vi "KE622x -- 2182 -A Set Digital Filter Type.vi"(0 "622x Resource In":refnum<visa-resource-name>, 1 "Check For SCPI Errors? (T)":bool=TRUE, 7 "Filter Type":T1=enum."Repeat", 11 "error in (no error)":errorcluster) -> (4 "622x Resource Out (dupl)":refnum<visa-resource-name>, 15 "error out":errorcluster)   [LabVIEW 2019, in "Keithley 622x.lvlib"]
uses:
  Keithley 622x.lvlib
  Typedefs/KE2182 -- Filter Type.ctl
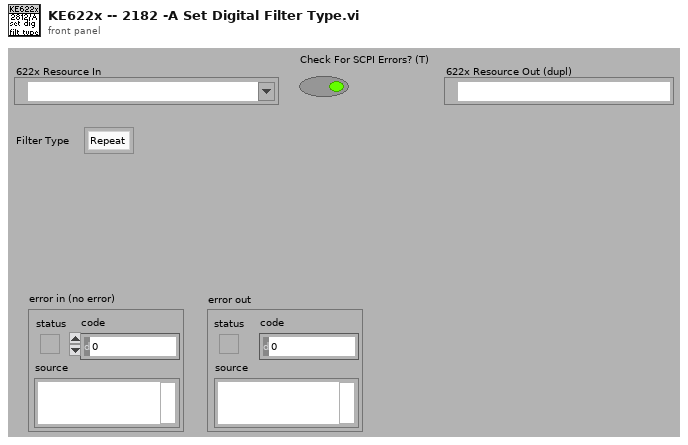
[diagram p1: front panel]
types:
  T1 = typedef "Keithley 622x.lvlib/KE2182 -- Filter Type.ctl" = enum16{"Moving", "Repeat"}
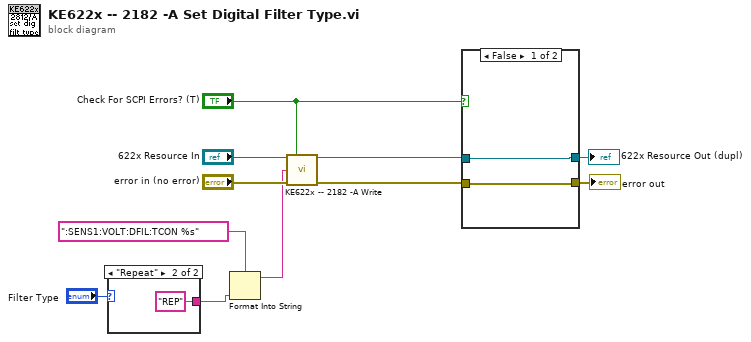
[diagram p0: block diagram]
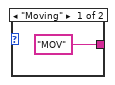
[diagram p2: hidden frame]
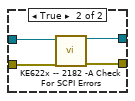
[diagram p3: hidden frame]
diagram:
  n1 = case shown="\"Repeat\"" "Filter Type" {
    tunnel: ["MOV" "REP"] -> w1
    frame "Moving" {
    }
    frame "Repeat" {
    }
  }
  n2 = Format Into String(format string=":SENS1:VOLT:DFIL:TCON %s", w1) -> (resulting string=w4:string)  [unwired: 2 in, 1 out]
  n3 = call "KE622x -- 2182 -A Write.vi"("Resource In"="622x Resource In", "Check For SCPI Errors? (T)"="Check For SCPI Errors? (T)", "2182-A Write String"=w4, "error in (no error)"="error in (no error)") -> ("Resource Out (dupl)"=w9:refnum<visa-resource-name>, "error out"=w3:errorcluster)  [unwired: 10 in]
  n4 = case shown="False" "Check For SCPI Errors? (T)" {
    tunnel: w9 -> [w15 w19]
    tunnel: w3 -> [w14 w18]
    tunnel: [w15 w17] -> w7
    tunnel: [w14 w16] -> w6
    frame False {
    }
    frame True {
      n5 = call "KE622x -- 2182 -A Check For SCPI Errors.vi"("VISA Resource In"=w19, "error in (no error)"=w18) -> ("VISA Resource Out (dupl)"=w17:refnum<visa-resource-name>, "error out"=w16:errorcluster)  [unwired: 10 in, 2 out]
    }
  }
  "622x Resource Out (dupl)" <- w7
  "error out" <- w6
